vi "JPL Arm Control.vi"(0 "Elevator Array":dbl, 7 "Joystick Boolean Inputs":T1, 11 "Actual Height":dbl) -> (4 "Arms Release":bool, 8 "Elevator Final Reference":dbl, 15 "Arms Closed":bool)   [LabVIEW 2014]
uses:
  <vilib>/functionblocks/Counter/Timer Off Delay/Timer Off Delay.vi
  <vilib>/functionblocks/FB Core/FB Core.xnode
  <vilib>/functionblocks/NI_FunctionBlock Libraries.lvlib
panel:
  out "Barrel Grab":bool
  out "Tote Grabbed":bool
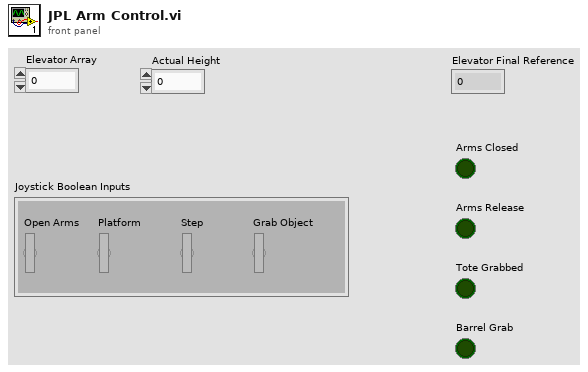
[diagram p1: front panel]
types:
  T1 = cluster{"Open Arms":bool, "Platform":bool, "Step":bool, "Grab Object":bool}
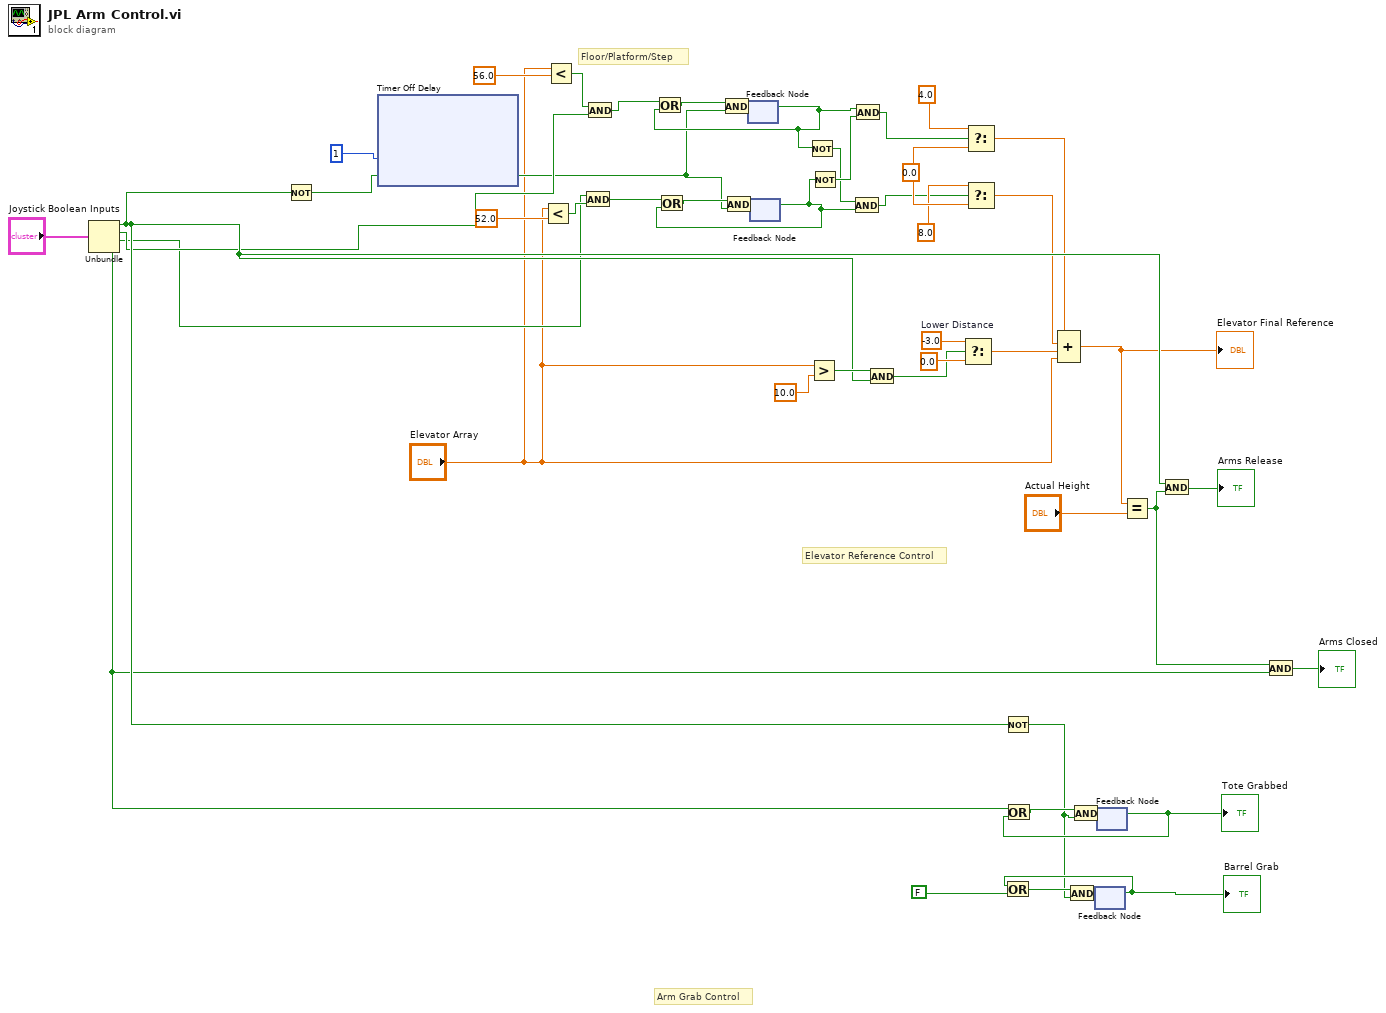
[diagram p0: block diagram]
diagram:
  w46 = 0.0
  w48 = -3.0  # Lower Distance
  # "Floor/Platform/Step"
  # "Arm Grab Control"
  # "Elevator Reference Control"
  n1 = Unbundle("Joystick Boolean Inputs") -> ("Open Arms"=w16:bool, "Platform"=w15:bool, "Step"=w14:bool, "Grab Object"=w6:bool)
  n2 = Not(x=w16) -> (.not. x?=w11:bool)
  n3 = xnode "Timer Off Delay"("preset time (ms)"=1, "input"=w11) -> ("output"=w10:bool)  [unwired: 1 in, 2 out]
  n4 = Less?(x="Elevator Array", y=52.0) -> (x < y?=w43:bool)
  n5 = Less?(x="Elevator Array", y=56.0) -> (x < y?=w41:bool)
  n6 = And(x=w14, y=w43) -> (x .and. y?=w25:bool)
  n7 = And(x=w41, y=w15) -> (x .and. y?=w26:bool)
  n8 = feedback #1() -> (w20:bool)  [unwired: 1 in]
  n9 = Or(x=w26, y=w20) -> (x .or. y?=w30:bool)
  n10 = And(x=w30, y=w10) -> (x .and. y?=w29:bool)
  n11 = feedback-in #1(w29) -> ()
  n12 = feedback #2() -> (w21:bool)  [unwired: 1 in]
  n13 = Or(x=w25, y=w21) -> (x .or. y?=w28:bool)
  n14 = And(x=w28, y=w10) -> (x .and. y?=w27:bool)
  n15 = feedback-in #2(w27) -> ()
  n16 = Not(x=w20) -> (.not. x?=w18:bool)
  n17 = Greater?(x="Elevator Array", y=10.0) -> (0:w38:bool)
  n18 = Not(x=w21) -> (.not. x?=w19:bool)
  n19 = And(x=w18, y=w21) -> (x .and. y?=w22:bool)
  n20 = And(x=w20, y=w19) -> (x .and. y?=w23:bool)
  n21 = And(x=w38, y=w16) -> (x .and. y?=w39:bool)
  n22 = Select(t=w48, s=w39, f=0.0) -> (s? t:f=w5:dbl)
  n23 = Select(t=4.0, s=w23, f=w46) -> (s? t:f=w1:dbl)
  n24 = Select(t=8.0, s=w22, f=w46) -> (s? t:f=w2:dbl)
  n25 = Not(x=w16) -> (.not. x?=w24:bool)
  n26 = Compound Arithmetic op=ADD(w1, w2, w5, "Elevator Array") -> (w3:dbl)
  "Elevator Final Reference" <- w3
  n27 = feedback #3() -> (w32:bool)  [unwired: 1 in]
  "Barrel Grab" <- w32
  n28 = Or(x=w32, y=FALSE) -> (x .or. y?=w36:bool)
  n29 = And(x=w36, y=w24) -> (x .and. y?=w33:bool)
  n30 = feedback-in #3(w33) -> ()
  n31 = feedback #4() -> (w31:bool)  [unwired: 1 in]
  "Tote Grabbed" <- w31
  n32 = Or(x=w6, y=w31) -> (x .or. y?=w35:bool)
  n33 = And(x=w35, y=w24) -> (x .and. y?=w34:bool)
  n34 = feedback-in #4(w34) -> ()
  n35 = Equal?(x=w3, y="Actual Height") -> (x = y?=w7:bool)
  n36 = And(x=w16, y=w7) -> (x .and. y?=→"Arms Release":bool)
  n37 = And(x=w7, y=w6) -> (x .and. y?=→"Arms Closed":bool)
